vi "Digilens DLP Gen2 UI .vi"(11 "TopLevel In":refnum<class "TopLevel.lvclass">) -> (3 "TopLevel Out":refnum<class "TopLevel.lvclass">)   [LabVIEW 2022 SP3, in "TopLevel.lvclass"] (continued)
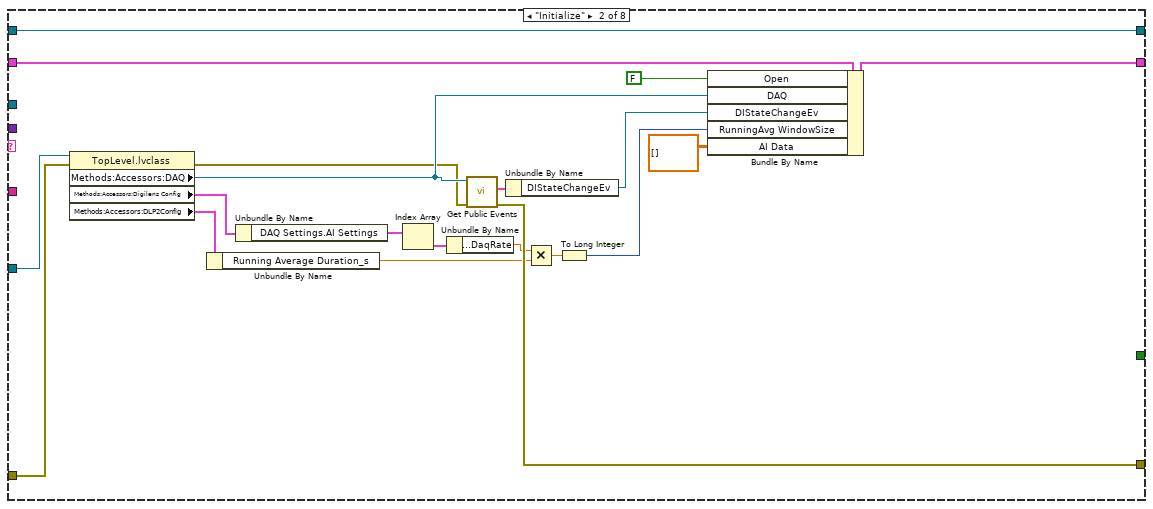
[diagram p3: hidden frame]
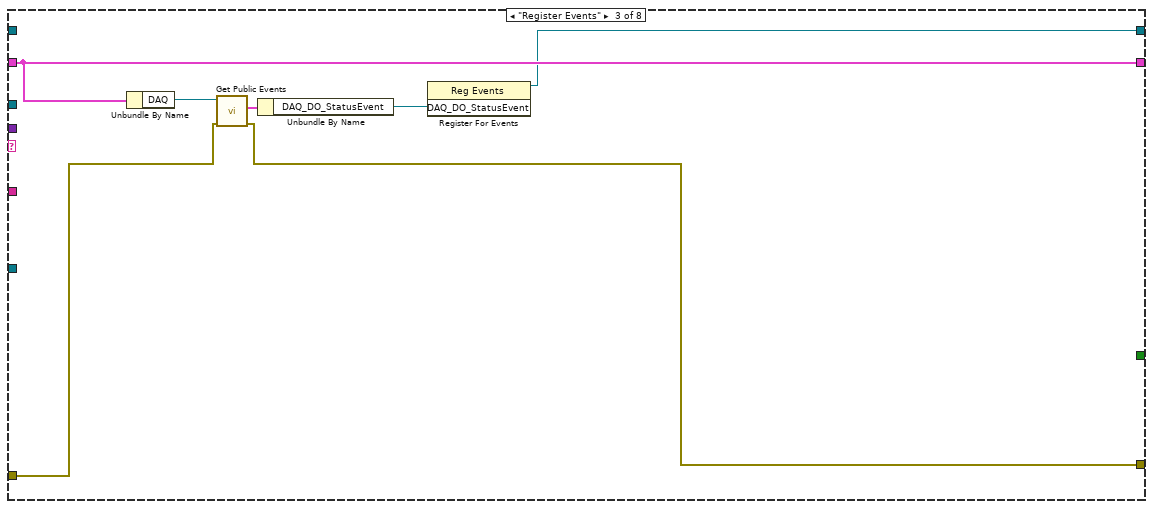
[diagram p4: hidden frame]
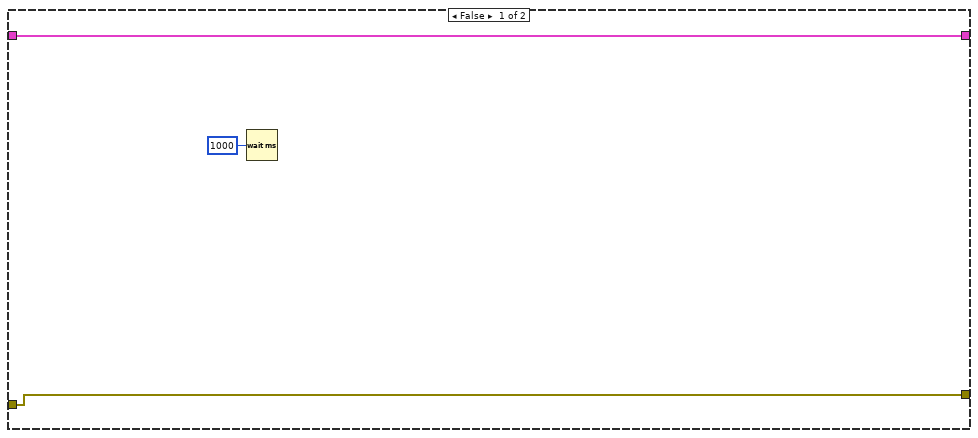
[diagram p5: hidden frame]
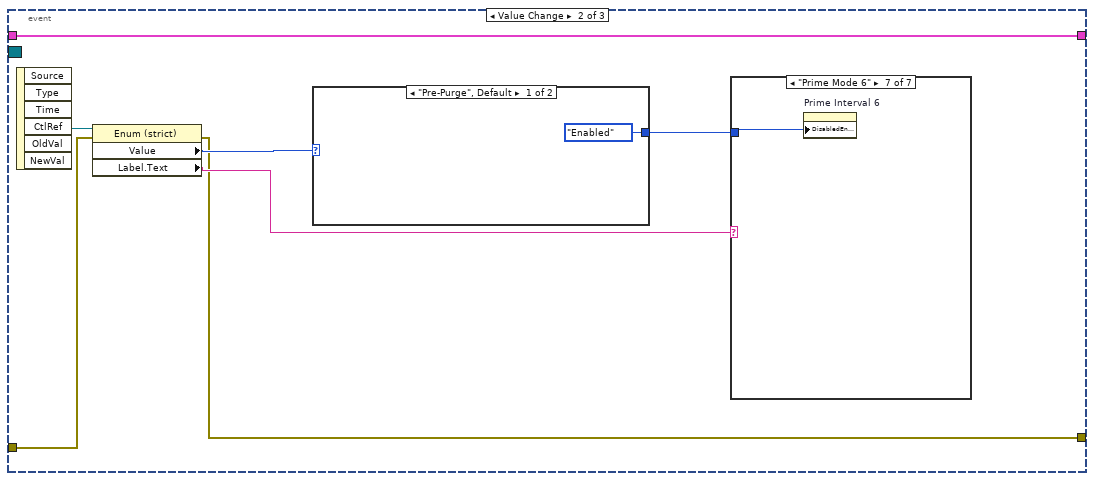
[diagram p7: hidden frame]
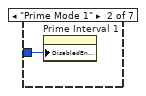
[diagram p9: hidden frame]
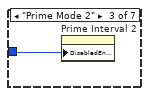
[diagram p10: hidden frame]
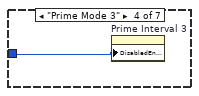
[diagram p11: hidden frame]
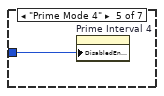
[diagram p12: hidden frame]
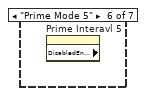
[diagram p13: hidden frame]
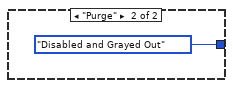
[diagram p14: hidden frame]
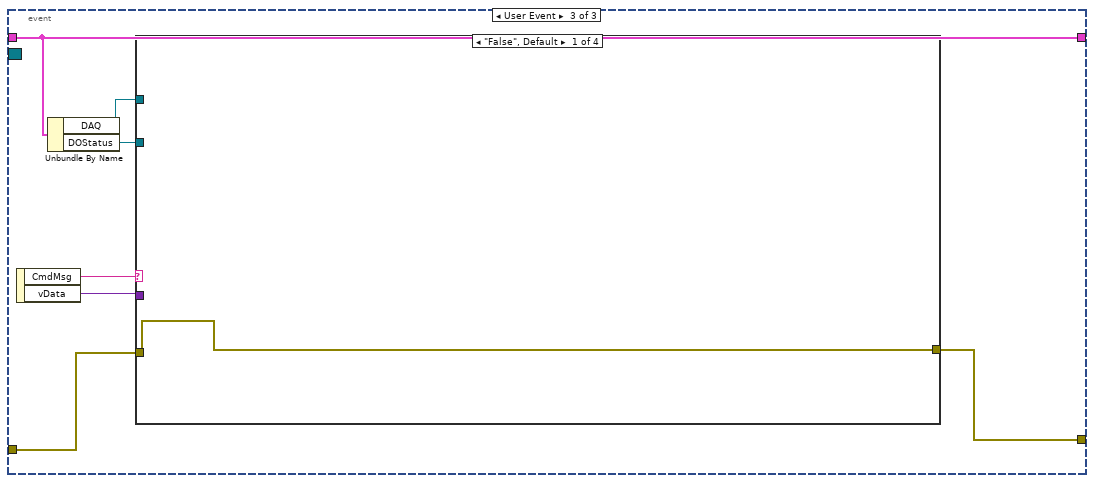
[diagram p15: hidden frame]
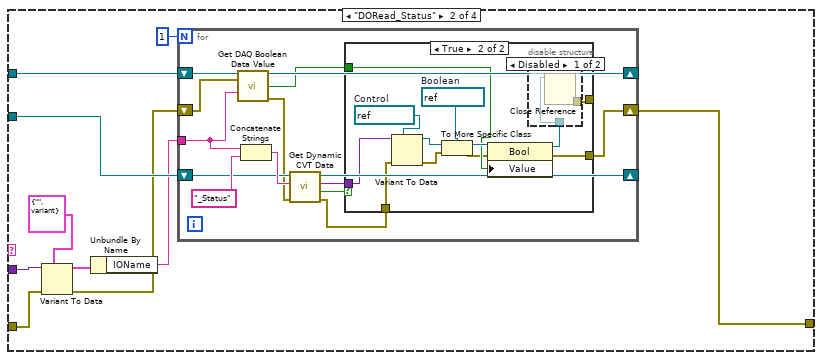
[diagram p16: hidden frame]
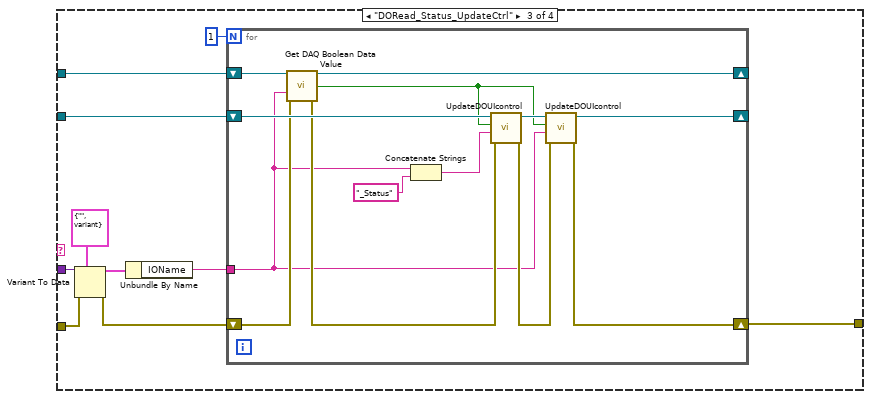
[diagram p19: hidden frame]
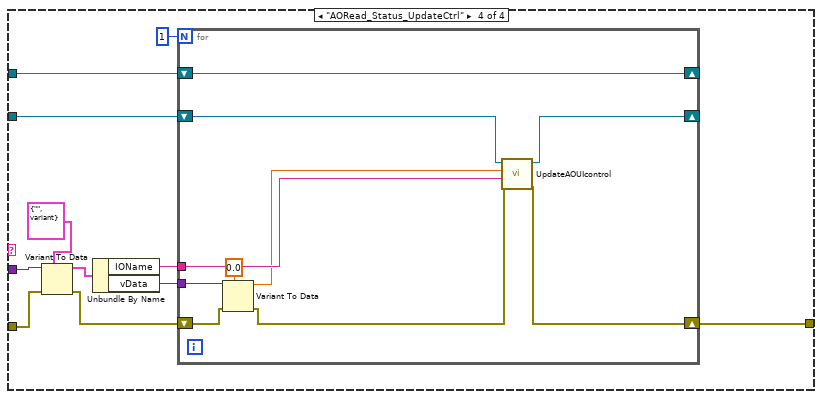
[diagram p20: hidden frame]
        n1718 = Format Into String(format string="%s", ICP1-AO_Channel_Names."Meniscus Vac Pump Speed" ("AO Channel")) -> (resulting string=w4719:string)  [unwired: 2 in, 1 out]
        n1719 = call "Set AO Data Value (manual mode).vi"("error in (no error)"=w4714, "Value"="Meniscus Vac Pump Speed", "AO IOName"=w4719, "DAQ"=w4720) -> ("error out"=w4715:errorcluster)  [unwired: 6 in, 1 out]
        n1720 = Bundle By Name(cluster=w4716, "PersistentData.Meniscus Vac Pump Speed"="Meniscus Vac Pump Speed") -> (w4713:T77)
        n1721 = call <vilib>:"Add State(s) to Queue__JKI_lib_State_Machine.vi"("State(s) in Front (\"\")"="Data: Write to Persistent File" ("State(s) in Front (\"\")"), "State(s) in (\"\")"=w4710) -> ("States Out"=w4711:string)  [unwired: 13 in]
      }
      frame "---------Mesniscus Pressure----------" {
      }
      frame "Set Meniscus Pressure" {
        n1722 = case shown="\"R2\"" w4728 {
          tunnel: [ICP1-AO_Channel_Names."Meniscus Pressure Set - R1" ("AO Channel") ICP1-AO_Channel_Names."Meniscus Pressure Set - R2" ("AO Channel") ICP1-AO_Channel_Names."Meniscus Pressure Set - R3" ("AO Channel") ICP1-AO_Channel_Names."Meniscus Pressure Set - R4" ("AO Channel") ICP1-AO_Channel_Names."Meniscus Pressure Set - R5" ("AO Channel") ICP1-AO_Channel_Names."Meniscus Pressure Set - R6" ("AO Channel")] -> w4738
          tunnel: ["Meniscus Pressure Set - R1" "Meniscus Pressure Set - R2" "Meniscus Pressure Set - R3" "Meniscus Pressure Set - R4" "Meniscus Pressure Set - R5" "Meniscus Pressure Set - R6"] -> w4737
          tunnel: w4732 -> [w4746 w4749 w4753 w4758 w4761 w4765]
          tunnel: [w4744 w4748 w4752 w4757 w4760 w4764] -> w4733
          frame "R1", Default {
            n1723 = Bundle By Name(cluster=w4746, "PersistentData.MiniscusPressure.Meniscus Pressure Set - R1"="Meniscus Pressure Set - R1") -> (w4744:T77)
          }
          frame "R2" {
            n1724 = Bundle By Name(cluster=w4749, "PersistentData.MiniscusPressure.Meniscus Pressure Set - R2"="Meniscus Pressure Set - R2") -> (w4748:T77)
          }
          frame "R3" {
            n1725 = Bundle By Name(cluster=w4753, "PersistentData.MiniscusPressure.Meniscus Pressure Set - R3"="Meniscus Pressure Set - R3") -> (w4752:T77)
          }
          frame "R4" {
            n1726 = Bundle By Name(cluster=w4758, "PersistentData.MiniscusPressure.Meniscus Pressure Set - R4"="Meniscus Pressure Set - R4") -> (w4757:T77)
          }
          frame "R5" {
            n1727 = Bundle By Name(cluster=w4761, "PersistentData.MiniscusPressure.Meniscus Pressure Set - R5"="Meniscus Pressure Set - R5") -> (w4760:T77)
          }
          frame "R6" {
            n1728 = Bundle By Name(cluster=w4765, "PersistentData.MiniscusPressure.Meniscus Pressure Set - R6"="Meniscus Pressure Set - R6") -> (w4764:T77)
          }
        }
        n1729 = Unbundle By Name(w4733) -> ("DAQ"=w4741:refnum<class "DAQ.lvclass">)
        n1730 = Format Into String(format string="%s", error in=w4734, w4738) -> (resulting string=w4740:string, error out=w4736:errorcluster)  [unwired: 1 in]
        n1731 = call "Set AO Data Value (manual mode).vi"("error in (no error)"=w4736, "Value"=w4737, "AO IOName"=w4740, "DAQ"=w4741) -> ("error out"=w4735:errorcluster)  [unwired: 6 in, 1 out]
        n1732 = call <vilib>:"Add State(s) to Queue__JKI_lib_State_Machine.vi"("State(s) in Front (\"\")"="Data: Write to Persistent File" ("State(s) in Front (\"\")"), "State(s) in (\"\")"=w4730) -> ("States Out"=w4731:string)  [unwired: 13 in]
      }
      frame "Set Meniscus Pressure Value" {
        n1733 = call <vilib>:"Parse State Queue__JKI_lib_State_Machine.vi"("State Queue"=w4768) -> ("Current State"=w4771:string, "Arguments"=w4773:string)  [unwired: 12 in, 1 out]
        n1734 = Fract/Exp String To Number(string=w4773) -> (number=w4770:dbl)  [unwired: 3 in, 1 out]
        n1735 = Scan From String(input string=w4771, default 1=PrinterHeads--Enum."-1" ("Head")) -> (output 1=w4769:T18)  [unwired: 3 in, 3 out]
        n1736 = case shown="\"5\"" w4769 {
          tunnel: [ICP1-AO_Channel_Names."None" ("AO Channel") ICP1-AO_Channel_Names."Meniscus Pressure Set - R1" ("AO Channel") ICP1-AO_Channel_Names."Meniscus Pressure Set - R2" ("AO Channel") ICP1-AO_Channel_Names."Meniscus Pressure Set - R3" ("AO Channel") ICP1-AO_Channel_Names."Meniscus Pressure Set - R4" ("AO Channel") ICP1-AO_Channel_Names."Meniscus Pressure Set - R5" ("AO Channel") ICP1-AO_Channel_Names."Meniscus Pressure Set - R6" ("AO Channel")] -> w4783
          tunnel: [0.0 w4792 w4796 w4800 w4804 w4808 w4812] -> w4782
          tunnel: w4777 -> [w4790 w4794 w4798 w4802 w4806 w4810 w4814]
          tunnel: [w4790 w4793 w4797 w4801 w4805 w4809 w4813] -> w4778
          tunnel: w4770 -> [_ w4792 w4796 w4800 w4804 w4808 w4812]
          frame "-1", Default {
          }
          frame "1" {
            n1737 = Bundle By Name(cluster=w4794, "PersistentData.MiniscusPressure.Meniscus Pressure Set - R1"=w4792) -> (w4793:T77)
            n1738 = local write "Meniscus Pressure Set - R1"(w4792) -> ()
          }
          frame "2" {
            n1739 = Bundle By Name(cluster=w4798, "PersistentData.MiniscusPressure.Meniscus Pressure Set - R2"=w4796) -> (w4797:T77)
            n1740 = local write "Meniscus Pressure Set - R2"(w4796) -> ()
          }
          frame "3" {
            n1741 = Bundle By Name(cluster=w4802, "PersistentData.MiniscusPressure.Meniscus Pressure Set - R3"=w4800) -> (w4801:T77)
            n1742 = local write "Meniscus Pressure Set - R3"(w4800) -> ()
          }
          frame "4" {
            n1743 = local write "Meniscus Pressure Set - R4"(w4804) -> ()
            n1744 = Bundle By Name(cluster=w4806, "PersistentData.MiniscusPressure.Meniscus Pressure Set - R4"=w4804) -> (w4805:T77)
          }
          frame "5" {
            n1745 = Bundle By Name(cluster=w4810, "PersistentData.MiniscusPressure.Meniscus Pressure Set - R5"=w4808) -> (w4809:T77)
            n1746 = local write "Meniscus Pressure Set - R5"(w4808) -> ()
          }
          frame "6" {
            n1747 = local write "Meniscus Pressure Set - R6"(w4812) -> ()
            n1748 = Bundle By Name(cluster=w4814, "PersistentData.MiniscusPressure.Meniscus Pressure Set - R6"=w4812) -> (w4813:T77)
          }
        }
        n1749 = Unbundle By Name(w4778) -> ("DAQ"=w4786:refnum<class "DAQ.lvclass">)
        n1750 = Format Into String(format string="%s", error in=w4779, w4783) -> (resulting string=w4785:string, error out=w4781:errorcluster)  [unwired: 1 in]
        n1751 = call "Set AO Data Value (manual mode).vi"("error in (no error)"=w4781, "Value"=w4782, "AO IOName"=w4785, "DAQ"=w4786) -> ("error out"=w4780:errorcluster)  [unwired: 6 in, 1 out]
        n1752 = call <vilib>:"Add State(s) to Queue__JKI_lib_State_Machine.vi"("State(s) in Front (\"\")"="Data: Write to Persistent File" ("State(s) in Front (\"\")"), "State(s) in (\"\")"=w4775) -> ("States Out"=w4776:string)  [unwired: 13 in]
      }
      frame "---------Recirc Pump Flow---------" {
      }
      frame "-------Set Temperature----" {
      }
      frame "Set Head Temperature" {
        n1753 = call <vilib>:"Parse State Queue__JKI_lib_State_Machine.vi"("State Queue"=w4833) -> ("Current State"=w4830:string, "Arguments"=w4832:string)  [unwired: 12 in, 1 out]
        n1754 = Unbundle By Name(w4834) -> ("TopLevel out"=w4836:refnum<class "TopLevel.lvclass">)
        n1755 = Fract/Exp String To Number(string=w4832) -> (number=w4826:dbl)  [unwired: 3 in, 1 out]
        n1756 = Scan From String(input string=w4830, error in=w4828, default 1=PrinterHeads--Enum."-1" ("Head")) -> (error out=w4829:errorcluster, output 1=w4827:T18)  [unwired: 2 in, 2 out]
        n1757 = call-dynamic "SetHeadHeaterTemperature API.vi"("error in (no error)"=w4829, "SetPoint (deg)"=w4826, "Head"=w4827, "TopLevel in"=w4836) -> ("error out"=w4835:errorcluster)  [unwired: 6 in, 1 out]
        n1758 = case shown="\"-1\", Default" w4827 {
          tunnel: w4826 -> [_ w4840 w4841 w4842 w4843 w4844 w4845]
          frame "-1", Default {
          }
          frame "1" {
            n1759 = local write "Head1 TempSet"(w4840) -> ()
          }
          frame "2" {
            n1760 = local write "Head2 TempSet"(w4841) -> ()
          }
          frame "3" {
            n1761 = local write "Head3 TempSet"(w4842) -> ()
          }
          frame "4" {
            n1762 = local write "Head4 TempSet"(w4843) -> ()
          }
          frame "5" {
            n1763 = local write "Head 5 Act Temp"(w4844) -> ()
          }
          frame "6" {
            n1764 = local write "Head 6 Act Temp"(w4845) -> ()
          }
        }
      }
      frame "SetRecircPump" {
        n1765 = call <vilib>:"Parse State Queue__JKI_lib_State_Machine.vi"("State Queue"=w4859) -> ("Current State"=w4857:string, "Arguments"=w4849:string)  [unwired: 12 in, 1 out]
        n1766 = Unbundle By Name(w4860) -> ("DAQ"=w4852:refnum<class "DAQ.lvclass">)
        n1767 = Scan From String(input string=w4849, default 1=FALSE) -> (output 1=w4846:bool)  [unwired: 3 in, 3 out]
        n1768 = Scan From String(input string=w4857, error in=w4856, default 1=PrinterHeads--Enum."-1" ("Head")) -> (output 1=w4855:T18)  [unwired: 2 in, 3 out]
        n1769 = case shown="\"-1\", Default" w4855 {
          tunnel: w4846 -> [_ w4866 w4868 w4870 w4872 w4874 w4876]
          tunnel: [ICP2-DO_Channel_Names."None" ("DO Channel") ICP2-DO_Channel_Names."Recirc Pump On - R1" ("DO Channel") ICP2-DO_Channel_Names."Recirc Pump On - R2" ("DO Channel") ICP2-DO_Channel_Names."Recirc Pump On - R3" ("DO Channel") ICP2-DO_Channel_Names."Recirc Pump On - R4" ("DO Channel") ICP2-DO_Channel_Names."Recirc Pump On - R5" ("DO Channel") ICP2-DO_Channel_Names."Recirc Pump On - R6" ("DO Channel")] -> w4847
          frame "-1", Default {
          }
          frame "1" {
            n1770 = local write "Recirc Pump On - R1"(w4866) -> ()
          }
          frame "2" {
            n1771 = local write "Recirc Pump On - R2"(w4868) -> ()
          }
          frame "3" {
            n1772 = local write "Recirc Pump On - R3"(w4870) -> ()
          }
          frame "4" {
            n1773 = local write "Recirc Pump On - R4"(w4872) -> ()
          }
          frame "5" {
            n1774 = local write "Recirc Pump On - R5"(w4874) -> ()
          }
          frame "6" {
            n1775 = local write "Recirc Pump On - R6"(w4876) -> ()
          }
        }
        n1776 = Format Into String(format string="%s", w4847) -> (resulting string=w4854:string, error out=w4850:errorcluster)  [unwired: 2 in]
        n1777 = call "Set DO State (manual mode).vi"("error in (no error)"=w4850, "State"=w4846, "DO IOName"=w4854, "DAQ"=w4852) -> ("error out"=w4851:errorcluster)  [unwired: 6 in, 1 out]
      }
    }
  }
  "TopLevel Out" <- w14
  n1778 = while {
    tunnel: w1 -> [w4883]
    shift-right: [w4887] -> _
    shift-left: w11 -> [w4889]
    shift-right: [w4884] -> _
    shift-left: w8 -> [w4885]
    tunnel: w5 -> [w4881]
    shift-right: [w4879] -> _
    shift-left: _ -> [w4878]
    stop <- w4890 stop-if-true
    n1779 = call <vilib>:"Get Next Queued State with vData.vi"("queue in"=w4883, "error in (no error)"=w4889) -> ("vData out"=w4886:variant, "queue out"=w4882:refnum<queue>, "Next State"=w4880:string, "queued msg"=w4877:string, "error out"=w4888:errorcluster)  [unwired: 7 in, 2 out]
    n1780 = case shown="\"\", \"EventHandler\", \"Idle\"" w4880 {
      tunnel: [_ _ _ _ _ _ _ TRUE] -> w4890
      tunnel: w4888 -> [w4893 w4909 w4917 w4925 w5099 w5108 w5137 w5143]
      tunnel: [w4893 w4905 w4918 w4924 errorcluster {"status"=FALSE, "code"=0, "source"=""} ("error out") w5107 w5136 w5143] -> w4887
      tunnel: w4886 -> [_ _ _ _ _ w5109 _ _]
      tunnel: w4885 -> [w4892 w4913 w4920 w4923 w5098 w5106 w5140 w5142]
      tunnel: [w4892 w4912 w4920 w4922 w5098 w5105 w5135 w5142] -> w4884
      tunnel: w4882 -> [_ _ _ _ _ _ w5139 _]
      tunnel: w4881 -> [_ w4910 _ _ _ _ _ _]
      tunnel: [w4891 w4908 w4914 w4921 w5097 w5104 w5133 w5141] -> w4879
      tunnel: w4878 -> [w4891 w4908 _ w4921 w5097 w5104 w5133 w5141]
      tunnel: w4877 -> [_ _ _ _ _ w5103 _ _]
      frame Default {
      }
      frame "Initialize" {
        n1781 = property class="TopLevel.lvclass"(reference=w4910, error in=w4909) -> (error out=w4906:errorcluster, "Methods:Accessors:DAQ"=w4907:refnum<class "DAQ.lvclass">, "Methods:Accessors:Digilens Config"=w4902:T51, "Methods:Accessors:DLP2Config"=w4899:T35)  [unwired: 1 out]
        n1782 = Unbundle By Name(w4899) -> ("Running Average Duration_s"=w4897:dbl)
        n1783 = Unbundle By Name(w4902) -> ("DAQ Settings.AI Settings"=w4901:T58[])
        n1784 = Index Array(array=w4901) -> (element=w4900:T58)  [unwired: 1 in]
        n1785 = Unbundle By Name(w4900) -> ("AI InstSettings.DaqRate"=w4898:dbl)
        n1786 = call "Get Public Events.vi"("error in (no error)"=w4906, "DAQ"=w4907) -> ("error out"=w4905:errorcluster, "PublicEvents"=w4904:T102)  [unwired: 7 in, 1 out]
        n1787 = Unbundle By Name(w4904) -> ("DIStateChangeEv"=w4903:refnum<user-event>)
        n1788 = Multiply(x=w4898, y=w4897) -> (x*y=w4896:dbl)
        n1789 = To Long Integer(number=w4896) -> (32bit integer=w4895:i32)
        n1790 = Bundle By Name(cluster=w4913, "Open"=FALSE, "DAQ"=w4907, "DIStateChangeEv"=w4903, "RunningAvg WindowSize"=w4895, "AI Data"=dbl[][] []) -> (w4912:T17)
      }
      frame "Register Events" {
        n1791 = Unbundle By Name(w4920) -> ("DAQ"=w4919:refnum<class "DAQ.lvclass">)
        n1792 = call "Get Public Events.vi"("error in (no error)"=w4917, "DAQ"=w4919) -> ("error out"=w4918:errorcluster, "PublicEvents"=w4916:T102)  [unwired: 7 in, 1 out]
        n1793 = Unbundle By Name(w4916) -> ("DAQ_DO_StatusEvent"=w4915:refnum<user-event>)
        n1794 = register-events(w4915) -> (reference out=w4914:refnum<event-registration>)  [unwired: 2 in, 1 out]
      }
      frame "", "EventHandler", "Idle" {
        n1795 = event shown="[0] Timeout" {
          selector: w4921 -> [_ _ _]
          dyn-events: _ -> [_ _ _]
          timeout: 1 -> [_ _ _]
          tunnel: w4923 -> [w4930 w4994 w5012]
          tunnel: w4925 -> [w4928 w4993 w5007]
          tunnel: [w4927 w4992 w5009] -> w4924
          tunnel: [w4931 w4994 w5012] -> w4922
          event Timeout {
            n1796 = event-data() -> ()  [unwired: 1 in, 3 out]
            n1797 = Unbundle By Name(w4930) -> ("Open"=w4929:bool)
            n1798 = case shown="True" w4929 {
              tunnel: w4930 -> [w4934 w4977]
              tunnel: [w4934 w4941] -> w4931
              tunnel: w4928 -> [w4933 w4936]
              tunnel: [w4933 w4936] -> w4927
              frame False {
                n1799 = Wait (ms)(milliseconds to wait=u32 1000) -> ()  [unwired: 1 out]
              }
              frame True {
                n1800 = Unbundle By Name(w4977) -> ("AI Data"=w4946:dbl[][], "RunningAvg WindowSize"=w4948:i32, "DAQ"=w4976:refnum<class "DAQ.lvclass">)
                n1801 = Array Size(array=w4946) -> (size(s)=w4950:i32[])
                n1802 = Index Array(array=w4950) -> (element=w4949:i32)  [unwired: 1 in]
                n1803 = call "Get DAQ AI ScanArray Data.vi"("DAQ"=w4976, "DataName"="AITask_1_AIScanArray", "error in (no error)"=w4936) -> ("DAQ"=w4967:refnum<class "DAQ.lvclass">, "AI ScanArray"=w4944:dbl[], "error out"=w4974:errorcluster)  [unwired: 8 in, 2 out]
                "AI ScanArray" <- w4944
                n1804 = Greater Or Equal?(x=w4949, y=w4948) -> (x >= y?=w4947:bool)
                n1805 = call "Get DAQ DI ScanArray Data.vi"("DAQ"=w4967, "error in (no error)"=w4936) -> ("DI ScanArray"=w4965:bool[], "error out"=w4966:errorcluster)  [unwired: 9 in, 3 out]
                n1806 = case shown="True" w4947 {
                  tunnel: w4946 -> [w4987 w4990]
                  tunnel: [w4987 w4988] -> w4945
                  frame False {
                  }
                  frame True {
                    n1807 = Delete From Array(array=w4990, index (row)=0) -> (array with subset deleted=w4988:dbl[][])  [unwired: 2 in, 1 out]
                  }
                }
                n1808 = Index Array(array=w4965) -> (element #1=→"SW - Ink Valve - R1":bool, element #2=→"SW - Ink Valve - R2":bool, element #3=→"SW - Ink Valve - R3":bool, element #4=→"SW - Ink Valve - R4":bool, element #5=→"SW - Ink Valve - R5":bool, element #6=→"SW - Ink Valve - R6":bool, element #7=→"SW - Purge - R1":bool, element #8=→"SW - Purge - R2":bool, element #9=→"SW - Purge - R3":bool, element #10=→"SW - Purge - R4":bool, element #11=→"SW - Purge - R5":bool, element #12=→"SW - Purge - R6":bool, element #13=→"SW - COVER INPUT SIDE":bool, element #14=→"SW - COVER OUTPUT SIDE":bool)  [unwired: 14 in]
                n1809 = flat-sequence {
                  tunnel: w4974 -> [_]
                  tunnel: w4966 -> [_]
                  tunnel: [errorcluster {"status"=FALSE, "code"=0, "source"=""} ("error out")] -> _
                  frame #0 {
                  }
                }
                n1810 = Insert Into Array(array=w4945, new element=w4944) -> (w4940:dbl[][])  [unwired: 2 in]
                n1811 = Bundle By Name(cluster=w4977, "AI Data"=w4940) -> (w4941:T17)
                n1812 = for {
                  N: 6 -> [_]
                  tunnel: w4940 -> [w4986]
                  tunnel: [w4983] -> w4942 mode=indexing
                  i -> [w4985]
                  n1813 = Index Array(array=w4986, index (col)=w4985) -> (element=w4984:dbl[])  [unwired: 1 in]
                  n1814 = call-poly <vilib>:"Mean.vi"("X"=w4984) -> ("mean"=w4983:dbl)  [unwired: 1 out]
                }
                n1815 = call "Get PrimeTimer Q.vi"("error in (no error)"=w4936) -> ("error out"=w4939:errorcluster, "ElementData[]"=w4938:variant[], "ElementNames[]"=w4937:string[])  [unwired: 7 in, 1 out]
                n1816 = Index Array(array=w4942) -> (element #1=→"Meniscus Pressure Read - R1":dbl, element #2=→"Meniscus Pressure Read - R2":dbl, element #3=→"Meniscus Pressure Read - R3":dbl, element #4=→"Meniscus Pressure Read - R4":dbl, element #5=→"Meniscus Pressure Read - R5":dbl, element #6=→"Meniscus Pressure Read - R6":dbl)  [unwired: 6 in]
                n1817 = flat-sequence {
                  tunnel: w4939 -> [w4979]
                  tunnel: w4938 -> [w4982]
                  tunnel: w4937 -> [_]
                  tunnel: [w4978] -> w4935
                  frame #0 {
                    n1818 = Index Array(array=w4982) -> (element=w4981:variant)  [unwired: 1 in]
                    n1819 = Variant To Data(error in=w4979, type=0, Variant=w4981) -> (data=w4978:i32)  [unwired: 1 out]
                  }
                }
                "HeadPrimeTimer" <- w4935
              }
            }
          }
          event Value Change {
            n1820 = event-data() -> ("CtlRef"=w4998:refnum<vi>)  [unwired: 1 in, 5 out]
            n1821 = property class="Enum (strict)"(reference=w4998, error in=w4993) -> (error out=w4992:errorcluster, "Value"=w4997:T13, "Label.Text"=w4996:string)  [unwired: 1 out]
            n1822 = case shown="\"Pre-Purge\", Default" w4997 {
              tunnel: [T45."Enabled" ("Disabled") T45."Disabled and Grayed Out" ("Disabled")] -> w4995
              frame "Pre-Purge", Default {
              }
              frame "Purge" {
              }
            }
            n1823 = case shown="\"Prime Mode 6\"" w4996 {
              tunnel: w4995 -> [_ w4999 w5000 w5001 w5002 _ w5003]
              frame "False", Default {
              }
              frame "Prime Mode 1" {
                n1824 = property on="Prime Interval 1" class="DigNum (strict)"("DisabledEnum"=w4999) -> ()  [unwired: 2 in, 2 out]
              }
              frame "Prime Mode 2" {
                n1825 = property on="Prime Interval 2" class="DigNum (strict)"("DisabledEnum"=w5000) -> ()  [unwired: 2 in, 2 out]
              }
              frame "Prime Mode 3" {
                n1826 = property on="Prime Interval 3" class="DigNum (strict)"("DisabledEnum"=w5001) -> ()  [unwired: 2 in, 2 out]
              }
              frame "Prime Mode 4" {
                n1827 = property on="Prime Interval 4" class="DigNum (strict)"("DisabledEnum"=w5002) -> ()  [unwired: 2 in, 2 out]
              }
              frame "Prime Mode 5" {
                n1828 = property on="Prime Interavl 5" class="DigNum (strict)" props=["DisabledEnum"]() -> ()  [unwired: 2 in, 3 out]
              }
              frame "Prime Mode 6" {
                n1829 = property on="Prime Interval 6" class="DigNum (strict)"("DisabledEnum"=w5003) -> ()  [unwired: 2 in, 2 out]
              }
            }
          }
          event User Event {
            n1830 = event-data() -> ("CmdMsg"=w5006:string, "vData"=w5008:variant)  [unwired: 1 in]
            n1831 = Unbundle By Name(w5012) -> ("DAQ"=w5011:refnum<class "DAQ.lvclass">, "DOStatus"=w5010:T16)
            n1832 = case shown="\"False\", Default" w5006 {
              tunnel: w5011 -> [_ w5023 w5062 w5086]
              tunnel: w5010 -> [_ w5022 w5061 w5085]
              tunnel: [w5013 w5021 w5060 w5084] -> w5009
              tunnel: w5008 -> [_ w5019 w5056 w5082]
              tunnel: w5007 -> [w5013 w5018 w5053 w5081]
              frame "False", Default {
              }
              frame "DORead_Status" {
                n1833 = Variant To Data(error in=w5018, type=T101 {"IOName"="", "vData"=variant} ("IOCtrlUpdate"), Variant=w5019) -> (data=w5015:T101, error out=w5017:errorcluster)
                n1834 = Unbundle By Name(w5015) -> ("IOName"=w5014:string)
                n1835 = for {
                  N: 1 -> [_]
                  shift-right: [w5030] -> w5021
                  shift-left: w5017 -> [w5027]
                  shift-right: [w5028] -> _
                  shift-left: w5023 -> [w5029]
                  shift-right: [w5034] -> _
                  shift-left: w5022 -> [w5035]
                  tunnel: w5014 -> [w5024]
                  n1836 = call "Get DAQ Boolean Data Value.vi"("DAQ"=w5029, "Name"=w5024, "error in (no error)"=w5027) -> ("DAQ"=w5028:refnum<class "DAQ.lvclass">, "Value"=w5025:bool, "error out"=w5026:errorcluster)  [unwired: 10 in]
                  n1837 = Concatenate Strings(w5024, "_Status" ("string")) -> (w5036:string)
                  n1838 = call <vilib>:"Get Dynamic CVT Data.vi"("error in (no error)"=w5026, "DataName"=w5036, "dCVT DVR"=w5035) -> ("error out"=w5031:errorcluster, "found"=w5033:bool, "value"=w5032:variant, "dCVT DVR out"=w5034:T16)  [unwired: 5 in]
                  n1839 = case shown="True" w5033 {
                    tunnel: w5032 -> [_ w5050]
                    tunnel: w5031 -> [w5038 w5045]
                    tunnel: w5025 -> [_ w5043]
                    tunnel: [w5038 w5039] -> w5030
                    tunnel: [_ w5040] -> _
                    frame False {
                    }
                    frame True {
                      w5048 = refnum<vi> refnum  # Boolean
                      w5049 = refnum<vi> refnum  # Control
                      n1840 = Variant To Data(error in=w5045, type=w5049, Variant=w5050) -> (data=w5047:refnum<vi>, error out=w5046:errorcluster)
                      n1841 = To More Specific Class(target class=w5048, reference=w5047, error in=w5046) -> (specific class reference=w5044:refnum<vi>, error out=w5042:errorcluster)
                      n1842 = property class="Bool"(reference=w5044, error in=w5042, "Value"=w5043) -> (reference out=w5041:refnum<vi>, error out=w5039:errorcluster)
                      n1843 = disable-structure shown="Disabled" {
                        disable-tunnel: w5041 -> [w5052 _]
                        disable-tunnel: [w5051 _] -> w5040
                        frame Disabled {
                          n1844 = Close Reference(reference=w5052) -> (error out=w5051:errorcluster)  [unwired: 1 in]
                        }
                        frame Enabled {
                        }
                      }
                    }
                  }
                }
              }
              frame "DORead_Status_UpdateCtrl" {
                n1845 = Variant To Data(error in=w5053, type=T101 {"IOName"="", "vData"=variant} ("IOCtrlUpdate"), Variant=w5056) -> (data=w5058:T101, error out=w5054:errorcluster)
                n1846 = Unbundle By Name(w5058) -> ("IOName"=w5055:string)
                n1847 = for {
                  N: 1 -> [_]
                  shift-right: [w5065] -> w5060
                  shift-left: w5054 -> [w5070]
                  shift-right: [w5071] -> _
                  shift-left: w5062 -> [w5072]
                  shift-right: [w5067] -> _
                  shift-left: w5061 -> [w5073]
                  tunnel: w5055 -> [w5063]
                  n1848 = call "Get DAQ Boolean Data Value.vi"("DAQ"=w5072, "Name"=w5063, "error in (no error)"=w5070) -> ("DAQ"=w5071:refnum<class "DAQ.lvclass">, "Value"=w5064:bool, "error out"=w5069:errorcluster)  [unwired: 10 in]
                  n1849 = Concatenate Strings(w5063, "_Status" ("string")) -> (w5074:string)
                  n1850 = call "UpdateDOUIcontrol.vi"("error in (no error)"=w5069, "String"=w5074, "Value"=w5064, "Data Value Reference in"=w5073) -> ("error out"=w5066:errorcluster, "Data Value Reference out"=w5068:T16)  [unwired: 6 in]
                  n1851 = call "UpdateDOUIcontrol.vi"("error in (no error)"=w5066, "String"=w5063, "Value"=w5064, "Data Value Reference in"=w5068) -> ("error out"=w5065:errorcluster, "Data Value Reference out"=w5067:T16)  [unwired: 6 in]
                }
              }
              frame "AORead_Status_UpdateCtrl" {
                n1852 = Variant To Data(error in=w5081, type=T101 {"IOName"="", "vData"=variant} ("IOCtrlUpdate"), Variant=w5082) -> (data=w5078:T101, error out=w5080:errorcluster)
                n1853 = Unbundle By Name(w5078) -> ("IOName"=w5077:string, "vData"=w5076:variant)
                n1854 = for {
                  N: 1 -> [_]
                  shift-right: [w5089] -> w5084
                  shift-left: w5080 -> [w5093]
                  shift-right: [w5096] -> _
                  shift-left: w5086 -> [w5096]
                  shift-right: [w5091] -> _
                  shift-left: w5085 -> [w5092]
                  tunnel: w5077 -> [w5088]
                  tunnel: w5076 -> [w5095]
                  n1855 = Variant To Data(error in=w5093, type=0.0, Variant=w5095) -> (data=w5087:dbl, error out=w5090:errorcluster)
                  n1856 = call "UpdateAOUIcontrol.vi"("error in (no error)"=w5090, "String"=w5088, "Numeric"=w5087, "Data Value Reference in"=w5092) -> ("error out"=w5089:errorcluster, "Data Value Reference out"=w5091:T16)  [unwired: 6 in]
                }
              }
            }
          }
        }
      }
      frame "Error Handler" {
        n1857 = call <vilib>:"General Error Handler.vi"("error in (no error)"=w5099) -> ()  [unwired: 10 in, 5 out]
      }
      frame "UpdateSettings" {
        n1858 = call <vilib>:"Parse State Queue__JKI_lib_State_Machine.vi"("State Queue"=w5103) -> ("Current State"=w5102:string, "Arguments"=w5101:string)  [unwired: 12 in, 1 out]
        n1859 = case shown="\"DOStatusDict\"" w5102 {
          tunnel: w5109 -> [_ w5113 w5120 _]
          tunnel: w5108 -> [w5111 w5114 w5121 w5124]
          tunnel: [w5111 w5115 w5122 w5124] -> w5107
          tunnel: w5106 -> [w5110 w5116 w5123 w5131]
          tunnel: [w5110 w5116 w5118 w5130] -> w5105
          tunnel: w5101 -> [_ _ _ w5125]
          frame "False", Default {
          }
          frame "Configuration" {
            n1860 = Variant To Data(error in=w5114, type="placeholder", Variant=w5113) -> (error out=w5115:errorcluster)  [unwired: 1 out]
          }
          frame "DOStatusDict" {
            w5119 = T16 refnum  # DOStatus
            n1861 = Variant To Data(error in=w5121, type=w5119, Variant=w5120) -> (data=w5117:T16, error out=w5122:errorcluster)
            n1862 = Bundle By Name(cluster=w5123, "DOStatus"=w5117) -> (w5118:T17)
          }
          frame "DAQStarted" {
            n1863 = Equal?(x=w5125, y="TRUE") -> (x = y?=w5128:bool)
            n1864 = Scan From String(input string=w5125, default 1=FALSE ("x = y?")) -> (output 1=→"AI":bool)  [unwired: 3 in, 3 out]
            n1865 = Bundle By Name(cluster=w5131, "Open"=w5128) -> (w5130:T17)
          }
        }
      }
      frame "Macro: Exit" {
        n1866 = Bundle By Name(cluster=w5140, "Open"=FALSE, "AI Data"=dbl[][] []) -> (w5135:T17)
        n1867 = call <vilib>:"Add States to Queue using MultiLine String (no vData input).vi"("queue in"=w5139, "states in"="Quit", "error in"=w5137) -> ("error out"=w5136:errorcluster)  [unwired: 10 in, 2 out]
      }
      frame "Quit" {
      }
    }
  }
